vi "Read Positioner Name.vi"(8 "error in (no error)":errorcluster, 11 "Newport in":refnum<class "Newport.lvclass">) -> (0 "error out":errorcluster, 2 "Positioner Name":string, 3 "Newport out":refnum<class "Newport.lvclass">)   [LabVIEW 2018, in "Newport.lvlib" / "Newport.lvclass"]
uses:
  Newport.lvclass
  Newport.lvclass/Newport.ctl
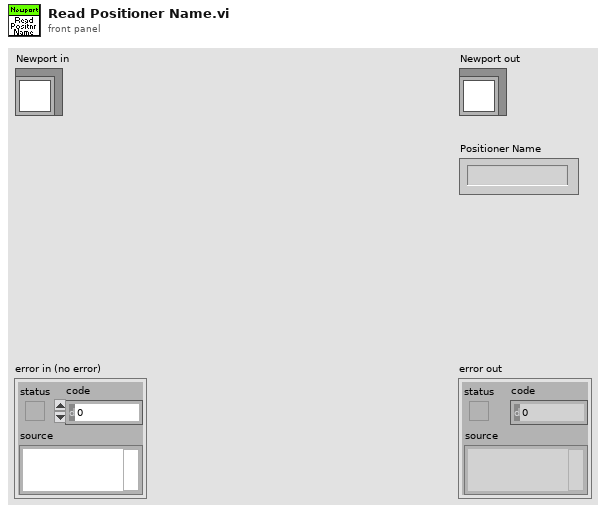
[diagram p1: front panel]
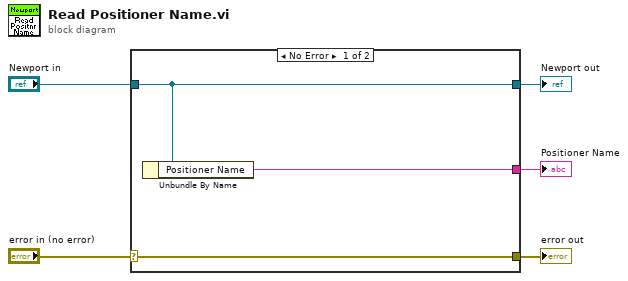
[diagram p0: block diagram]
diagram:
  n1 = case shown="No Error" "error in (no error)" {
    selector: "error in (no error)" -> [w8 w9]
    tunnel: [w8 w9] -> w4
    tunnel: [w7 w10] -> w2
    tunnel: "Newport in" -> [w7 w10]
    tunnel: [w6 _] -> w1
    frame No Error {
      n2 = Unbundle By Name(w7) -> ("Positioner Name"=w6:string)
    }
    frame Error {
    }
  }
  "error out" <- w4
  "Newport out" <- w2
  "Positioner Name" <- w1
